vi "MainTestCode.vi"() -> ()   [LabVIEW 2012]
uses:
  <userlib>/BotSpeak/VIs/SubVIs/BotSpeak_Globals.vi
panel:
  out "Cover":bool
  in  "Open":bool
  out "BotSpeak":string
  out "good?":bool
  in  "Console":bool
  out "Measured Response":string
  out "Expected Response":string
  out "Reply":string
  out "Script Sent":string
  out "Running":bool
  in  "Run All":bool
  in  "Run":bool
  in  "Done":bool
  in  "Test Codes":i32(listbox)=-1
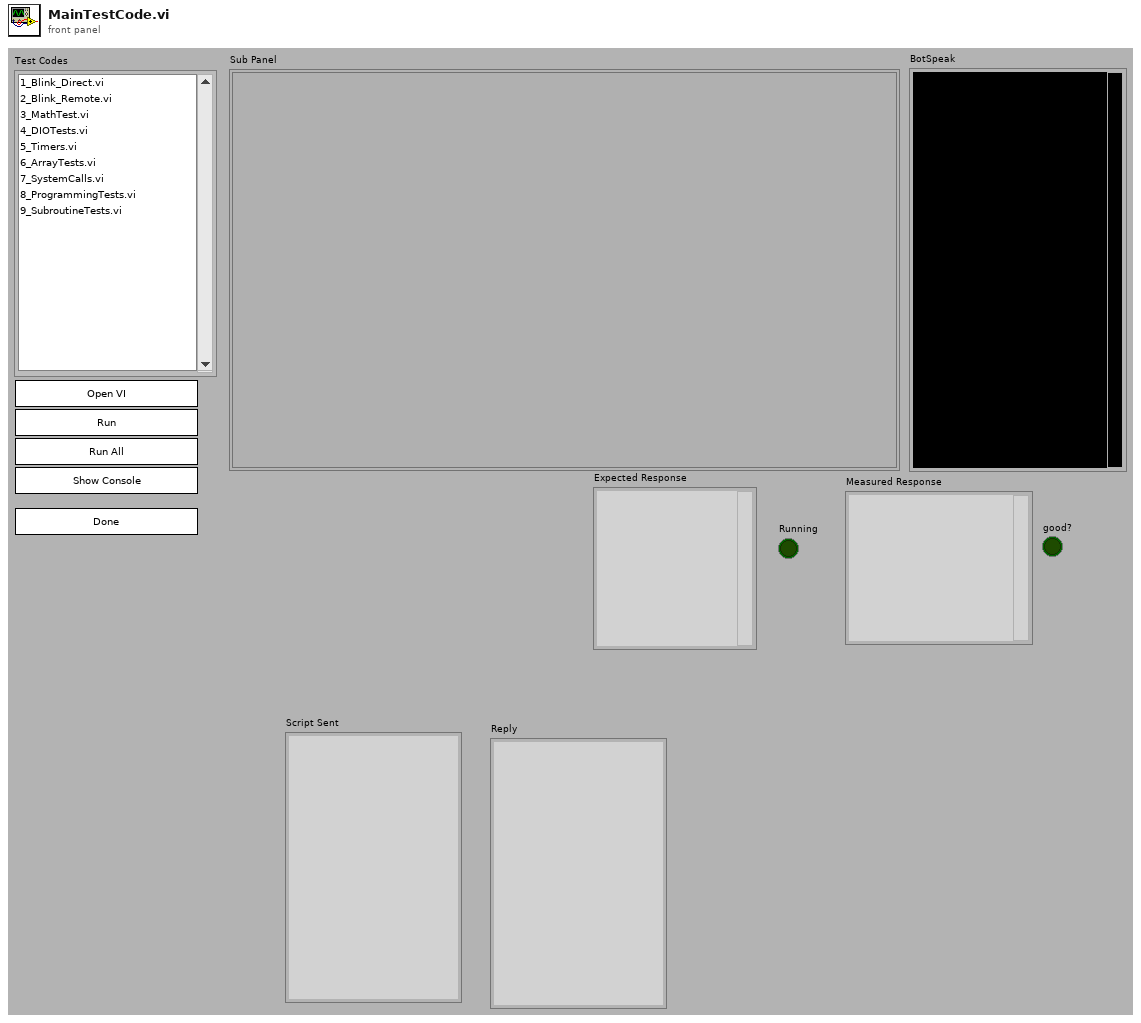
[diagram p1: front panel]
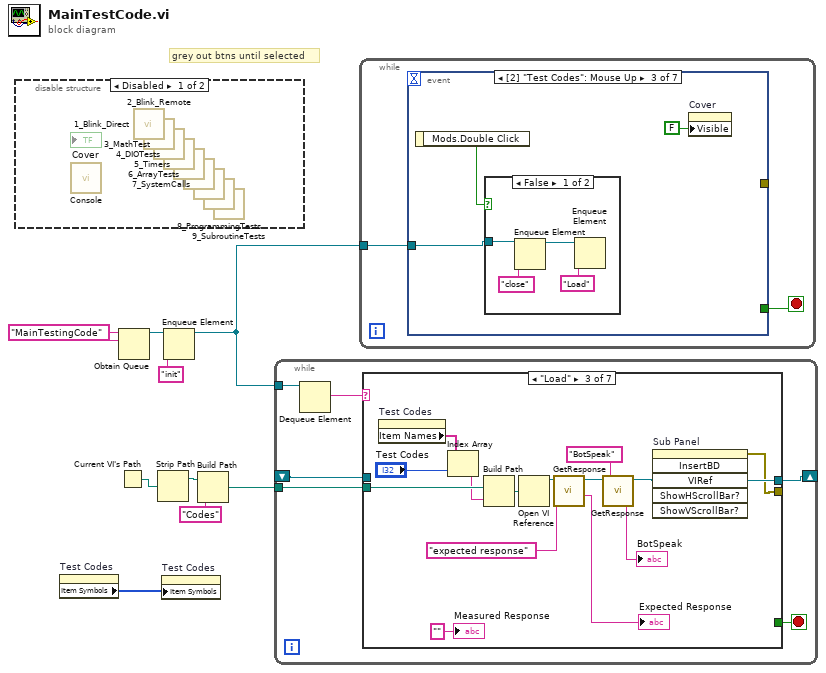
[diagram p0: block diagram]
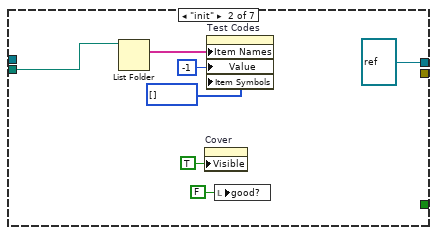
[diagram p4: hidden frame]
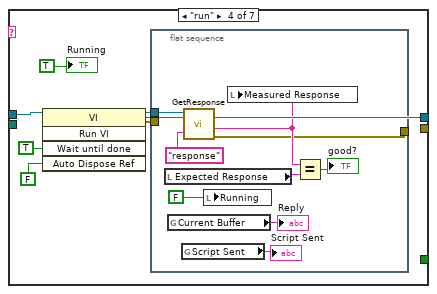
[diagram p5: hidden frame]
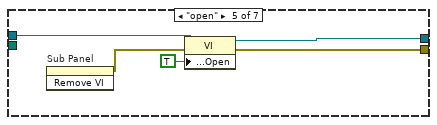
[diagram p6: hidden frame]
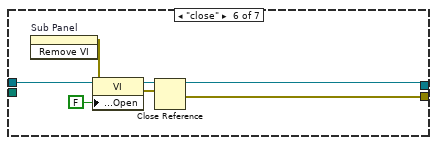
[diagram p7: hidden frame]
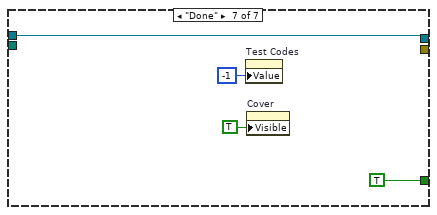
[diagram p8: hidden frame]
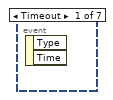
[diagram p9: hidden frame]
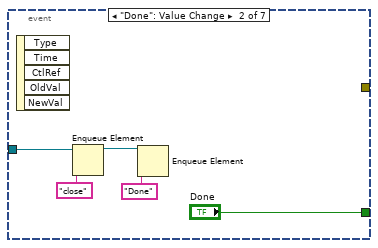
[diagram p10: hidden frame]
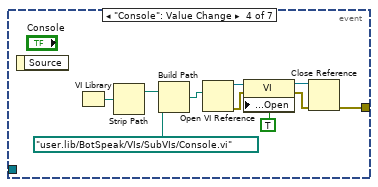
[diagram p12: hidden frame]
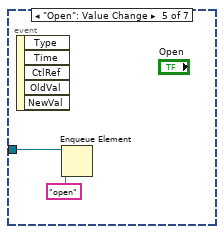
[diagram p13: hidden frame]
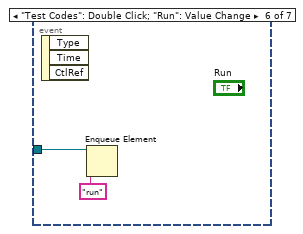
[diagram p14: hidden frame]
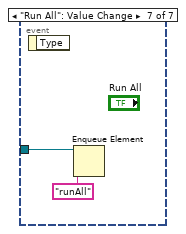
[diagram p15: hidden frame]
diagram:
  w9 = "MainTestingCode" ("name (unnamed)")
  # "grey out btns until selected"
  n1 = disable-structure shown="Disabled" {
    frame Disabled {
      n2 = call <userlib>:"Console.vi"() -> ()  [unwired: 4 in, 2 out]
      n3 = call <userlib>:"1_Blink_Direct.vi"() -> ()  [unwired: 12 in]
      n4 = call <userlib>:"2_Blink_Remote.vi"() -> ()  [unwired: 12 in]
      n5 = call <userlib>:"3_MathTest.vi"() -> ()  [unwired: 12 in]
      n6 = call <userlib>:"4_DIOTests.vi"() -> ()  [unwired: 12 in]
      n7 = call <userlib>:"5_Timers.vi"() -> ()  [unwired: 12 in]
      n8 = call <userlib>:"6_ArrayTests.vi"() -> ()  [unwired: 12 in]
      n9 = call <userlib>:"7_SystemCalls.vi"() -> ()  [unwired: 12 in]
      n10 = call <userlib>:"8_ProgrammingTests.vi"() -> ()  [unwired: 12 in]
      n11 = call <userlib>:"9_SubroutineTests.vi"() -> ()  [unwired: 12 in]
    }
    frame Enabled {
    }
  }
  n12 = property on="Test Codes" class="LstBox (strict)"() -> ("Item Symbols"=w1:i32[])  [unwired: 2 in, 2 out]
  n13 = Current VI's Path() -> (path=w4:path)
  n14 = Obtain Queue(name (unnamed)=w9, element data type=w9) -> (queue out=w8:refnum<queue>)  [unwired: 3 in, 2 out]
  n15 = Strip Path(path=w4) -> (stripped path=w5:path)  [unwired: 1 out]
  n16 = property on="Test Codes" class="LstBox (strict)"("Item Symbols"=w1) -> ()  [unwired: 2 in, 2 out]
  n17 = Enqueue Element(queue=w8, element="init") -> (queue out=w6:refnum<queue>)  [unwired: 2 in, 2 out]
  n18 = Build Path(base path=w5, name or relative path="Codes") -> (appended path=w2:path)
  n19 = while {
    tunnel: w6 -> [w15]
    tunnel: w2 -> [w13]
    shift-right: [w12] -> _
    shift-left: _ -> [w11]
    stop <- w14 stop-if-true
    n20 = Dequeue Element(queue=w15) -> (element=w10:string)  [unwired: 2 in, 3 out]
    n21 = case shown="\"Load\"" w10 {
      tunnel: [_ _ _ _ _ _ TRUE] -> w14
      tunnel: w13 -> [_ w21 w35 _ _ _ _]
      tunnel: [w16 refnum<vi> refnum ("vi reference") w27 w39 w56 w60 w66] -> w12
      tunnel: w11 -> [w16 _ _ w43 w57 w61 w66]
      tunnel: [_ _ w24 _ w53 w63 _] -> _
      frame Default {
      }
      frame "init" {
        n22 = List Folder(path=w21) -> (filenames=w23:string[])  [unwired: 3 in, 3 out]
        n23 = property on="Cover" class="Bool (strict)"("Visible"=TRUE) -> ()  [unwired: 2 in, 2 out]
        n24 = property on="Test Codes" class="LstBox (strict)"("Item Names"=w23, "Value"=-1 ("Test Codes"), "Item Symbols"=i32[] []) -> ()  [unwired: 2 in, 2 out]
        n25 = local write "good?"(FALSE ("good?")) -> ()
      }
      frame "Load" {
        n26 = property on="Test Codes" class="LstBox (strict)"() -> ("Item Names"=w37:string[])  [unwired: 2 in, 2 out]
        n27 = Index Array(array=w37, index="Test Codes") -> (element=w34:string)
        n28 = Build Path(base path=w35, name or relative path=w34) -> (appended path=w33:path)
        n29 = Open VI Reference(vi path=w33) -> (vi reference=w32:refnum<vi>)  [unwired: 5 in, 1 out]
        n30 = call <userlib>:"GetResponse.vi"("Name"="expected response", "vi reference in"=w32) -> ("value"=→"Expected Response":string, "vi reference out"=w28:refnum<vi>)  [unwired: 2 out]
        n31 = call <userlib>:"GetResponse.vi"("Name"="BotSpeak", "vi reference in"=w28) -> ("value"=→"BotSpeak":string, "vi reference out"=w27:refnum<vi>)  [unwired: 2 out]
        n32 = invoke on="Sub Panel" class="SubPanel" method="InsertBD"("VIRef"=w27) -> (error out=w24:errorcluster)  [unwired: 5 in, 5 out]
        "Measured Response" <- "" ("Measured Response")
      }
      frame "run" {
        n33 = invoke class="VI" method="Run VI"(reference=w43, "Wait until done"=TRUE ("Wait Until Done"), "Auto Dispose Ref"=FALSE ("Wait Until Done")) -> (reference out=w39:refnum<vi>, error out=w40:errorcluster)  [unwired: 2 in, 3 out]
        n34 = flat-sequence {
          tunnel: w40 -> [_]
          tunnel: w39 -> [w49]
          tunnel: [w44] -> _
          frame #0 {
            n35 = local read "Expected Response"() -> (w47:string)
            n36 = global read "BotSpeak_Globals.vi" "Current Buffer"() -> (→"Reply":string)
            n37 = global read "BotSpeak_Globals.vi" "Script Sent"() -> (→"Script Sent":string)
            n38 = call <userlib>:"GetResponse.vi"("Name"="response", "vi reference in"=w49) -> ("error out"=w44:errorcluster, "value"=w46:string)  [unwired: 2 out]
            n39 = local write "Running"(FALSE ("Running")) -> ()
            n40 = local write "Measured Response"(w46) -> ()
            n41 = Equal?(x=w46, y=w47) -> (x = y?=→"good?":bool)
          }
        }
        "Running" <- TRUE ("Running")
      }
      frame "open" {
        n42 = invoke on="Sub Panel" class="SubPanel" method="Remove VI"() -> (error out=w54:errorcluster)  [unwired: 3 in, 2 out]
        n43 = property class="VI"(reference=w57, error in=w54, "Front Panel.Open"=TRUE ("Front Panel Window:Open")) -> (reference out=w56:refnum<vi>, error out=w53:errorcluster)
      }
      frame "close" {
        n44 = invoke on="Sub Panel" class="SubPanel" method="Remove VI"() -> (error out=w59:errorcluster)  [unwired: 3 in, 2 out]
        n45 = property class="VI"(reference=w61, error in=w59, "Front Panel.Open"=FALSE ("Front Panel Window:Open")) -> (reference out=w60:refnum<vi>, error out=w58:errorcluster)
        n46 = Close Reference(reference=w60, error in (no error)=w58) -> (error out=w63:errorcluster)
      }
      frame "Done" {
        n47 = property on="Test Codes" class="LstBox (strict)"("Value"=-1 ("Test Codes")) -> ()  [unwired: 2 in, 2 out]
        n48 = property on="Cover" class="Bool (strict)"("Visible"=TRUE) -> ()  [unwired: 2 in, 2 out]
      }
    }
  }
  n49 = while {
    tunnel: w6 -> [w68]
    stop <- w69 stop-if-true
    n50 = event shown="[2] \"Test Codes\": Mouse Up" {
      selector: _ -> [_ _ _ _ _ _ _]
      dyn-events: _ -> [_ _ _ _ _ _ _]
      timeout: _ -> [_ _ _ _ _ _ _]
      tunnel: [_ "Done" _ _ _ _ _] -> w69
      tunnel: w68 -> [_ w71 w77 _ w92 w94 w96]
      tunnel: [_ _ _ w84 _ _ _] -> _
      event Timeout {
        n51 = event-data() -> ()  [unwired: 1 in, 2 out]
      }
      event "Done": Value Change {
        n52 = event-data() -> ()  [unwired: 1 in, 5 out]
        n53 = Enqueue Element(queue=w71, element="close") -> (queue out=w70:refnum<queue>)  [unwired: 2 in, 2 out]
        n54 = Enqueue Element(queue=w70, element="Done") -> ()  [unwired: 2 in, 3 out]
      }
      event "Test Codes": Mouse Up {
        n55 = event-data() -> ("Mods.Double Click"=w76:bool)  [unwired: 1 in]
        n56 = case shown="False" w76 {
          tunnel: w77 -> [w80 _]
          frame False {
            n57 = Enqueue Element(queue=w80, element="close") -> (queue out=w79:refnum<queue>)  [unwired: 2 in, 2 out]
            n58 = Enqueue Element(queue=w79, element="Load") -> ()  [unwired: 2 in, 3 out]
          }
          frame True {
          }
        }
        n59 = property on="Cover" class="Bool (strict)"("Visible"=FALSE) -> ()  [unwired: 2 in, 2 out]
      }
      event "Console": Value Change {
        n60 = event-data() -> ()  [unwired: 1 in, 1 out]
        n61 = VI Library() -> (path=w82:path)
        n62 = Strip Path(path=w82) -> (stripped path=w83:path)  [unwired: 1 out]
        n63 = Build Path(base path=w83, name or relative path=path "user.lib/BotSpeak/VIs/SubVIs/Console.vi") -> (appended path=w90:path)
        n64 = Open VI Reference(vi path=w90) -> (vi reference=w89:refnum<vi>, error out=w88:errorcluster)  [unwired: 5 in]
        n65 = property class="VI"(reference=w89, error in=w88, "Front Panel.Open"=TRUE ("Front Panel Window:Open")) -> (reference out=w86:refnum<vi>, error out=w87:errorcluster)
        n66 = Close Reference(reference=w86, error in (no error)=w87) -> (error out=w84:errorcluster)
      }
      event "Open": Value Change {
        n67 = event-data() -> ()  [unwired: 1 in, 5 out]
        n68 = Enqueue Element(queue=w92, element="open") -> ()  [unwired: 2 in, 3 out]
      }
      event "Test Codes": Double Click; "Run": Value Change {
        n69 = event-data() -> ()  [unwired: 1 in, 3 out]
        n70 = Enqueue Element(queue=w94, element="run") -> ()  [unwired: 2 in, 3 out]
      }
      event "Run All": Value Change {
        n71 = event-data() -> ()  [unwired: 1 in, 1 out]
        n72 = Enqueue Element(queue=w96, element="runAll") -> ()  [unwired: 2 in, 3 out]
      }
    }
  }
